vi "Read Save for version.vi"(8 "error in (no error)":errorcluster, 11 "Control.lvclass in":refnum<class "Control.lvclass">) -> (0 "error out":errorcluster, 2 "Save for version":string, 3 "Control.lvclass out":refnum<class "Control.lvclass">)   [LabVIEW 2013, in "Control.lvclass"]
doc: "Accessor VI for the control class"
uses:
  Control.lvclass
  Control.lvclass/Control.ctl
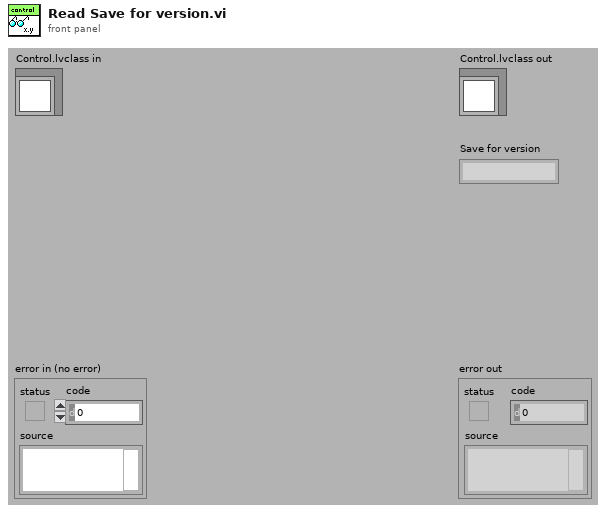
[diagram p1: front panel]
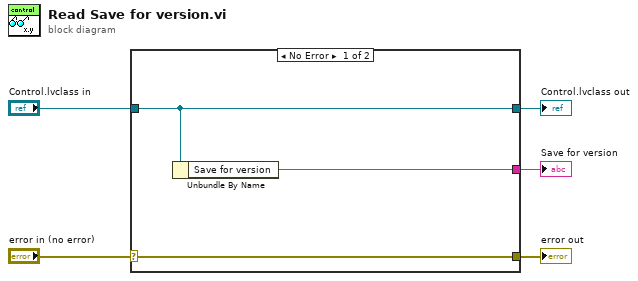
[diagram p0: block diagram]
diagram:
  n1 = case shown="No Error" "error in (no error)" {
    selector: "error in (no error)" -> [w8 w9]
    tunnel: [w8 w9] -> w4
    tunnel: [w7 w10] -> w2
    tunnel: "Control.lvclass in" -> [w7 w10]
    tunnel: [w6 _] -> w1
    frame No Error {
      n2 = Unbundle By Name(w7) -> ("Save for version"=w6:string)
    }
    frame Error {
    }
  }
  "error out" <- w4
  "Control.lvclass out" <- w2
  "Save for version" <- w1
